vi "Actor Core.vi"(8 "error in":errorcluster caption="错误输入", 11 "生命游戏 in":refnum<class "生命游戏.lvclass"> caption="操作者输入") -> (0 "error out":errorcluster caption="错误输出", 3 "Actor out":refnum<class "Actor.lvclass"> caption="操作者输出")   [LabVIEW 2015, in "生命游戏.lvlib" / "生命游戏.lvclass"]
doc: "(<B>Filename</B>: Actor Framework.lvlib:Actor.lvclass:Actor Core.vi)\n\nReceives messages to the actor, reacts to them, and initiates any error handling that may shut the actor down.\n\nDescendant classes may override this VI to append parallel tasks for the actor to complete while it handles messages.使用调用父方法节点实现重写。"
uses:
  <vilib>/ActorFramework/Actor/Actor.lvclass
  <vilib>/ActorFramework/Stop Msg/Stop Msg.lvclass
panel:
  in  "退出":bool
  in  "停止按钮":bool
  in  "开始":bool
  out "数组":bool[][](array[boolean])
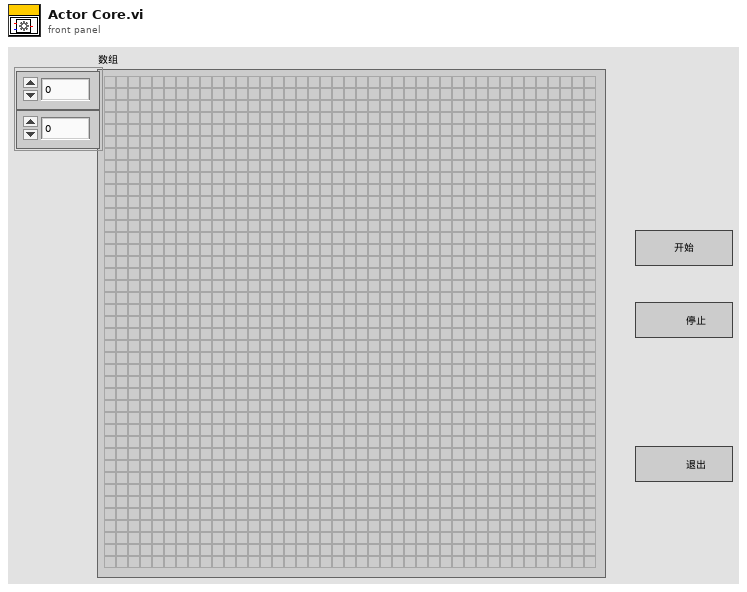
[diagram p1: front panel]
types:
  T1 = enum32{"Invalid", "Standard", "Closed", "Hidden", "Minimized", "Maximized"}
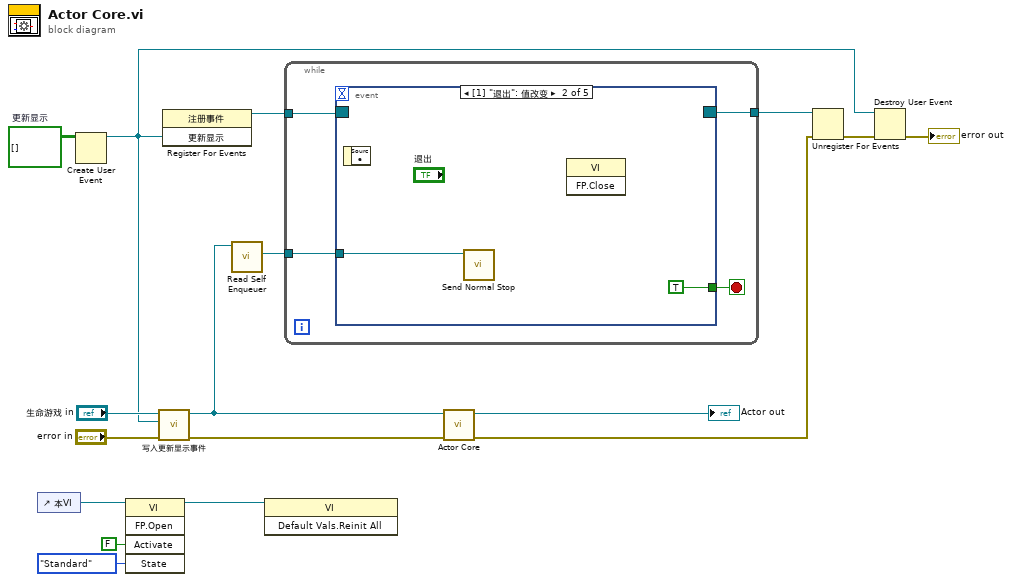
[diagram p0: block diagram]
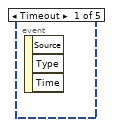
[diagram p2: hidden frame]
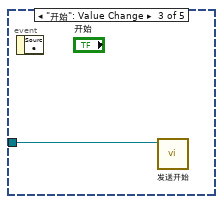
[diagram p3: hidden frame]
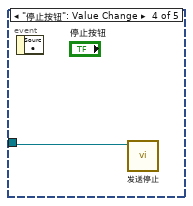
[diagram p4: hidden frame]
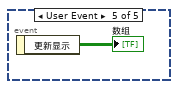
[diagram p5: hidden frame]
diagram:
  w15 = bool[][] []  # 更新显示
  n1 = control-ref of="本VI"() -> (w4:refnum<vi>)
  n2 = Create User Event(user event datatype=w15) -> (user event=w5:refnum<user-event>)  [unwired: 1 in, 1 out]
  n3 = invoke class="VI" method="FP.Open"(reference=w4, "Activate"=FALSE ("激活？"), "State"=T1."Standard" ("状态")) -> (reference out=w1:refnum<vi>)  [unwired: 2 in, 4 out]
  n4 = call "写入更新显示事件.vi"("error in (no error)"="error in", "更新显示事件"=w5, "生命游戏输入"="生命游戏 in") -> ("error out"=w8:errorcluster, "生命游戏输出"=w9:refnum<class "生命游戏.lvclass">)  [unwired: 7 in]
  n5 = register-events(w5) -> (reference out=w14:refnum<event-registration>)  [unwired: 2 in, 1 out]
  n6 = call <vilib>:"Read Self Enqueuer.vi"("Actor"=w9) -> ("Self Enqueuer"=w16:refnum<class "Message Enqueuer.lvclass">)  [unwired: 10 in]
  n7 = invoke class="VI" method="Default Vals.Reinit All"(reference=w1) -> ()  [unwired: 2 in, 3 out]
  n8 = while {
    tunnel: w16 -> [w21]
    tunnel: w14 -> [w19]
    tunnel: [w18] -> w13
    stop <- w20 stop-if-true
    n9 = event shown="[1] \"退出\": 值改变" {
      selector: w19 -> [_ _ _ _ _]
      dyn-events: [_ _ _ _ _] -> w18
      timeout: _ -> [_ _ _ _ _]
      tunnel: w21 -> [_ w23 w24 w25 _]
      tunnel: [_ TRUE _ _ _] -> w20
      event Timeout {
        n10 = event-data() -> ()  [unwired: 1 in, 3 out]
      }
      event "退出": Value Change {
        n11 = event-data() -> ()  [unwired: 1 in, 1 out]
        n12 = call <vilib>:"Send Normal Stop.vi"("Message Enqueuer"=w23) -> ()  [unwired: 10 in, 1 out]
        n13 = invoke class="VI" method="FP.Close"() -> ()  [unwired: 3 in, 3 out]
      }
      event "开始": Value Change {
        n14 = event-data() -> ()  [unwired: 1 in, 1 out]
        n15 = call "发送开始.vi"("Message Enqueuer"=w24) -> ()  [unwired: 9 in, 2 out]
      }
      event "停止按钮": Value Change {
        n16 = event-data() -> ()  [unwired: 1 in, 1 out]
        n17 = call "发送停止.vi"("Message Enqueuer"=w25) -> ()  [unwired: 9 in, 2 out]
      }
      event User Event {
        n18 = event-data() -> ("更新显示"=→"数组":bool[][])  [unwired: 1 in]
      }
    }
  }
  n19 = call-parent "Actor Core.vi"("error in"=w8, "Actor in"=w9) -> ("error out"=w12:errorcluster, "Actor out"=→"Actor out":refnum<class "Actor.lvclass">)  [unwired: 8 in]
  n20 = Unregister For Events(event registration refnum=w13, error in=w12) -> (error out=w11:errorcluster)
  n21 = Destroy User Event(user event=w5, error in=w11) -> (error out=→"error out":errorcluster)
